vi "Zero.vi"(8 "error in (no error)":errorcluster, 11 "TestActor in":refnum<class "TestActor.lvclass">) -> (0 "error out":errorcluster, 3 "TestActor out":refnum<class "TestActor.lvclass">)   [LabVIEW 2015, in "TestActor.lvlib" / "TestActor.lvclass"]
doc: "This VI sends an User event to reset the counter in the Actor Core to 0."
uses:
  TestActor.lvclass
  TestActor.lvclass/TestActor.ctl
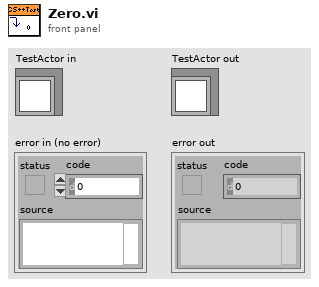
[diagram p1: front panel]
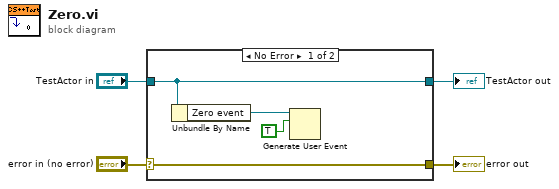
[diagram p0: block diagram]
diagram:
  n1 = case shown="No Error" "error in (no error)" {
    selector: "error in (no error)" -> [w8 w10]
    tunnel: [w8 w10] -> w3
    tunnel: [w7 w9] -> w1
    tunnel: "TestActor in" -> [w7 w9]
    frame No Error {
      n2 = Unbundle By Name(w7) -> ("Zero event"=w6:refnum<user-event>)
      n3 = Generate User Event(user event=w6, event data cluster=TRUE) -> ()  [unwired: 2 in, 2 out]
    }
    frame Error {
    }
  }
  "error out" <- w3
  "TestActor out" <- w1
